vi "Configure Digital Output.vi"(0 "VISA resource name":refnum<visa-resource-name>, 1 "Digital Output (1)":i16=1, 2 "Name (DIGIT OUT1)":string="DIGIT OUT1", 3 "Boost Percent Power (100.0)":dbl=100.0 format="%.2f", 4 "Boost Time Delay (30.0)":dbl=30.0 format="%.2f", 5 "error in (no error)":errorcluster {"code" format="%.0x"}, 6 "Unit Address (1)":i16=1, 7 "Compressor On % Power (0.0)":dbl format="%.2f", 8 "Function (0: Off)":u16(ring) items=["Off", "Event Output", "Complementary Output", "Control Output / Boost Heat", "Boost Cool", "Compressor"], 9 "Compressor Off % Power (0.0)":dbl format="%.2f", 11 "Compressor Off Delay (10.0)":dbl=10.0 format="%.2f", 13 "Compressor On Delay (30.0)":dbl=30.0 format="%.2f") -> (14 "VISA resource name out":refnum<visa-resource-name>, 19 "error out":errorcluster {"code" format="%.0x"})   [LabVIEW 2010]
doc: "This VI configures digital output."
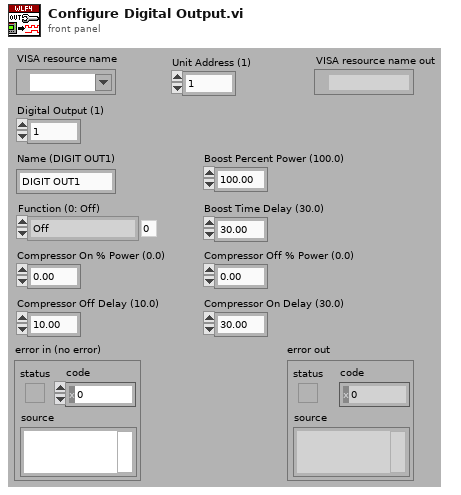
[diagram p1: front panel]
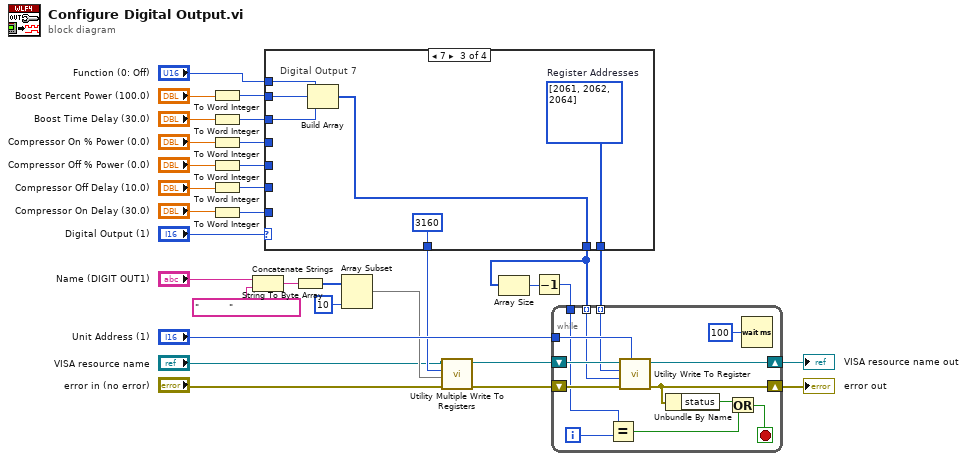
[diagram p0: block diagram]
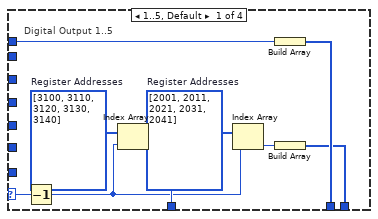
[diagram p2: hidden frame]
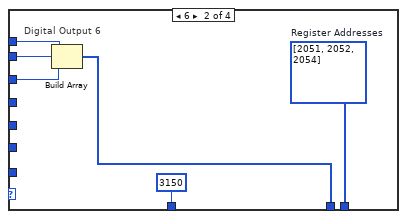
[diagram p3: hidden frame]
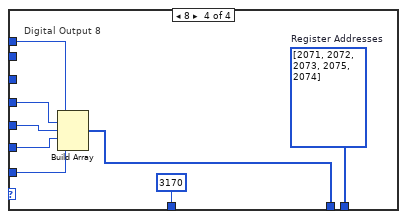
[diagram p4: hidden frame]
diagram:
  n1 = To Word Integer(number="Boost Percent Power (100.0)") -> (16bit integer=w1:i16)
  n2 = To Word Integer(number="Boost Time Delay (30.0)") -> (16bit integer=w3:i16)
  n3 = To Word Integer(number="Compressor On % Power (0.0)") -> (16bit integer=w4:i16)
  n4 = To Word Integer(number="Compressor Off % Power (0.0)") -> (16bit integer=w6:i16)
  n5 = To Word Integer(number="Compressor Off Delay (10.0)") -> (16bit integer=w17:i16)
  n6 = To Word Integer(number="Compressor On Delay (30.0)") -> (16bit integer=w16:i16)
  n7 = Concatenate Strings("Name (DIGIT OUT1)", "          " ("string")) -> (w26:string)
  n8 = case shown="7" "Digital Output (1)" {
    selector: "Digital Output (1)" -> [w35 _ _ _]
    tunnel: [w38 3150 3160 3170] -> w23
    tunnel: [w41 w42 w48 w54] -> w13
    tunnel: [w36 w46 w52 w60] -> w15
    tunnel: "Function (0: Off)" -> [w33 w45 w50 w59]
    tunnel: w1 -> [_ w44 w51 _]
    tunnel: w3 -> [_ w43 w49 _]
    tunnel: w4 -> [_ _ _ w55]
    tunnel: w6 -> [_ _ _ w58]
    tunnel: w17 -> [_ _ _ w57]
    tunnel: w16 -> [_ _ _ w56]
    frame 1..5, Default {
      w40 = i32[] [3100, 3110, 3120, 3130, 3140]  # Register Addresses
      w39 = i32[] [2001, 2011, 2021, 2031, 2041]  # Register Addresses
      # "Digital Output 1..5"
      n9 = Decrement(x=w35) -> (x-1=w34:i16)
      n10 = Index Array(array=w40, index=w34) -> (element=w38:i32)
      n11 = Index Array(array=w39, index=w34) -> (element=w37:i32)
      n12 = Build Array(w33) -> (w41:u16[])
      n13 = Build Array(w37) -> (w36:i32[])
    }
    frame 6 {
      w46 = i32[] [2051, 2052, 2054]  # Register Addresses
      # "Digital Output 6"
      n14 = Build Array(w45, w44, w43) -> (w42:u16[])
    }
    frame 7 {
      w52 = i32[] [2061, 2062, 2064]  # Register Addresses
      # "Digital Output 7"
      n15 = Build Array(w50, w51, w49) -> (w48:u16[])
    }
    frame 8 {
      w60 = i32[] [2071, 2072, 2073, 2075, 2074]  # Register Addresses
      # "Digital Output 8"
      n16 = Build Array(w59, w55, w58, w57, w56) -> (w54:u16[])
    }
  }
  n17 = String To Byte Array(string=w26) -> (unsigned byte array=w27:u8[])
  n18 = Array Subset(array=w27, length=10) -> (w25:u8[])  [unwired: 1 in]
  n19 = call "Utility Multiple Write To Registers.vi"("error in (no error)"="error in (no error)", "Array Of Data"=w25, "Register Address (0)"=w23, "VISA resource name"="VISA resource name") -> ("error out"=w9:errorcluster, "VISA resource name out"=w10:refnum<visa-resource-name>)  [unwired: 6 in]
  n20 = Array Size(array=w13) -> (size(s)=w14:i32)
  n21 = Decrement(x=w14) -> (x-1=w12:i32)
  n22 = while {
    tunnel: "Unit Address (1)" -> [w74]
    shift-right: [w71] -> w32
    shift-left: w10 -> [w73]
    shift-right: [w69] -> w31
    shift-left: w9 -> [w72]
    tunnel: w13 -> [w63] mode=indexing
    tunnel: w15 -> [w62] mode=indexing
    tunnel: w12 -> [w64]
    i -> [w66]
    stop <- w67 stop-if-true
    n23 = Equal?(x=w64, y=w66) -> (x = y?=w65:bool)
    n24 = call "Utility Write To Register.vi"("Unit Address (1)"=w74, "error in (no error)"=w72, "Data (0)"=w63, "Register Address (0)"=w62, "VISA resource name"=w73) -> ("error out"=w69:errorcluster, "VISA resource name out"=w71:refnum<visa-resource-name>)  [unwired: 5 in]
    n25 = Unbundle By Name(w69) -> ("status"=w68:bool)
    n26 = Or(x=w68, y=w65) -> (x .or. y?=w67:bool)
    n27 = Wait (ms)(milliseconds to wait=u32 100) -> ()  [unwired: 1 out]
  }
  "error out" <- w31
  "VISA resource name out" <- w32
